vi "Boolean Crossing (DBL).vi"(2 "initialize":bool, 3 "direction":enum16{"either", "false-true", "true-false"}(ring), 5 "input point":bool) -> (1 "crossing":bool)   [LabVIEW 2020, in "NI_AdvCtrl_nonlinear.lvlib"]
doc: "LabVIEW no longer supports this VI. You can obtain similar functionality by installing the LabVIEW Simulation Module.\n\nDetects boolean crossings of boolean input points. The user can choose from three different detectors, either, true-false, and false-true."
uses:
  <vilib>/addons/control/advanced/NI_AdvCtrl_nonlinear.lvlib
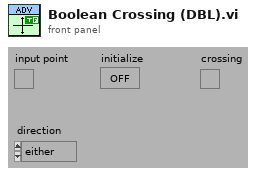
[diagram p1: front panel]
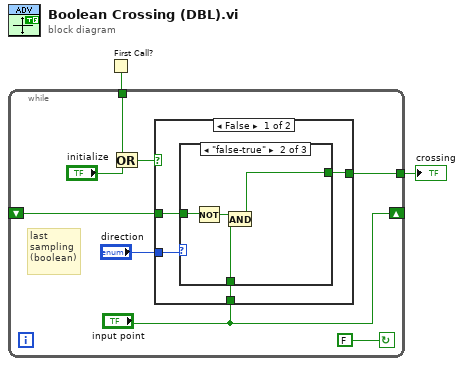
[diagram p0: block diagram]
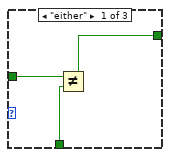
[diagram p2: hidden frame]
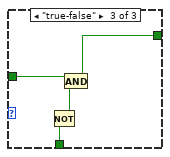
[diagram p3: hidden frame]
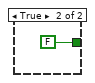
[diagram p4: hidden frame]
diagram:
  n1 = First Call?() -> (First Call?: T/F=w1:bool)
  n2 = while {
    tunnel: w1 -> [w4]
    tunnel: [w10] -> w2
    shift-left: _ -> [w8]
    shift-right: ["input point"] -> _
    stop <- FALSE continue-if-true
    # "last\nsampling\n(boolean)"
    n3 = Or(x=w4, y="initialize") -> (x .or. y?=w5:bool)
    n4 = case shown="False" w5 {
      tunnel: [w11 FALSE] -> w10
      tunnel: "direction" -> [w14 _]
      tunnel: w8 -> [w13 _]
      tunnel: "input point" -> [w12 _]
      frame False {
        n5 = case shown="\"false-true\"" w14 {
          tunnel: w13 -> [w17 w20 w22]
          tunnel: w12 -> [w16 w18 w24]
          tunnel: [w15 w21 w25] -> w11
          frame "either" {
            n6 = Not Equal?(x=w17, y=w16) -> (x != y?=w15:bool)
          }
          frame "false-true" {
            n7 = Not(x=w20) -> (.not. x?=w19:bool)
            n8 = And(x=w19, y=w18) -> (x .and. y?=w21:bool)
          }
          frame "true-false" {
            n9 = Not(x=w24) -> (.not. x?=w23:bool)
            n10 = And(x=w22, y=w23) -> (x .and. y?=w25:bool)
          }
        }
      }
      frame True {
      }
    }
  }
  "crossing" <- w2
